vi "extract_trace.vi"(8 "error in (no error)":errorcluster, 9 "sub-pixels":i32=1, 10 "start index":i32, 11 "ImageCollection in":refnum<class "ImageCollection.lvclass">) -> (0 "error out":errorcluster, 2 "trace":sgl[](graph))   [LabVIEW 2010]
uses:
  common/classes/ImageCollection/ImageCollection/ImageCollection.lvclass
  common/classes/Image/Image/Image.lvclass
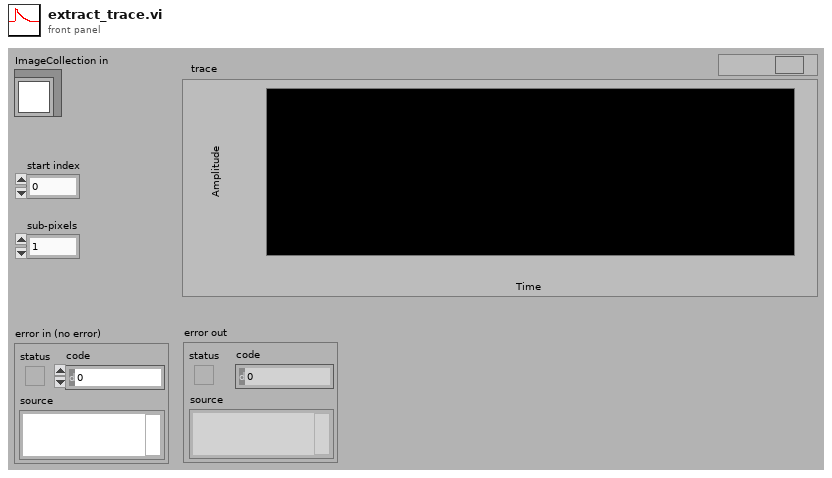
[diagram p1: front panel]
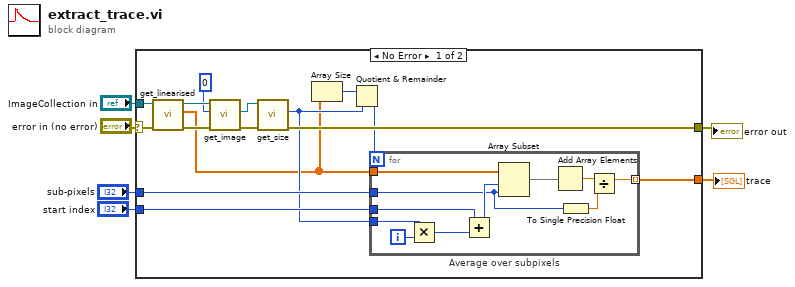
[diagram p0: block diagram]
diagram:
  n1 = case shown="No Error" "error in (no error)" {
    selector: "error in (no error)" -> [w21 w33]
    tunnel: "ImageCollection in" -> [w20 _]
    tunnel: "start index" -> [w19 _]
    tunnel: [w13 w33] -> w3
    tunnel: "sub-pixels" -> [w11 _]
    tunnel: [w9 _] -> w1
    frame No Error {
      n2 = call "get_linearised.vi"("error in (no error)"=w21, "ImageCollection in"=w20) -> ("error out"=w16:errorcluster, "pixels"=w7:sgl[], "ImageCollection out"=w18:refnum<class "ImageCollection.lvclass">)  [unwired: 7 in]
      n3 = call-dynamic "get_image.vi"("error in (no error)"=w16, "index"=0, "ImageCollection in"=w18) -> ("error out"=w14:errorcluster, "Image.lvclass"=w15:refnum<class "Image.lvclass">)  [unwired: 6 in, 1 out]
      n4 = call-dynamic "get_size.vi"("error in (no error)"=w14, "Image in"=w15) -> ("error out"=w13:errorcluster, "x resolution"=w8:i32)  [unwired: 2 in, 6 out]
      n5 = Array Size(array=w7) -> (size(s)=w12:i32)
      n6 = Quotient & Remainder(x=w12, y=w8) -> (floor(x/y)=w10:i32)  [unwired: 1 out]
      n7 = for "Average over subpixels" {
        N: w10 -> [_]
        tunnel: w7 -> [w30]
        tunnel: w19 -> [w22]
        tunnel: w8 -> [w31]
        tunnel: w11 -> [w24]
        tunnel: [w25] -> w9 mode=indexing
        i -> [w32]
        n8 = Multiply(x=w31, y=w32) -> (x*y=w23:i32)
        n9 = Add(x=w22, y=w23) -> (x+y=w29:i32)
        n10 = Array Subset(array=w30, index=w29, length=w24) -> (w28:sgl[])
        n11 = Add Array Elements(numeric array=w28) -> (sum=w27:sgl)
        n12 = To Single Precision Float(number=w24) -> (single precision float=w26:sgl)
        n13 = Divide(x=w27, y=w26) -> (x/y=w25:sgl)
      }
    }
    frame Error {
    }
  }
  "error out" <- w3
  "trace" <- w1
